vi "ConmonTest.vi"() -> ()   [LabVIEW 2020]
panel:
  out "index":i32
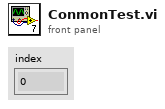
[diagram p1: front panel]
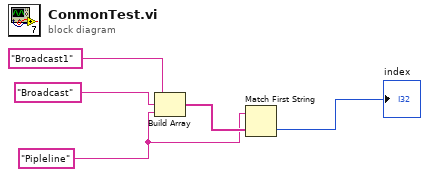
[diagram p0: block diagram]
diagram:
  w1 = "Pipleline" ("y")
  n1 = Build Array("Broadcast1" ("x"), "Broadcast" ("x"), w1) -> (w5:string[])
  n2 = Match First String(2:w5, 3:w1) -> (0:→"index":i32)  [unwired: 1 out]
